vi "Emballage_BDD_GPAO_V_ARTICLE_NOS_ARTtoINDEX.vi"(0 "codification":string, 5 "suffixe":string, 9 "clc_designation":string, 11 "error in (no error)":errorcluster) -> (2 "SUFFIXE":string, 3 "NB_PIECE_EMB":string, 4 "données":string[][](array[string]), 6 "id_article":string, 8 "INDICE_REV":string, 10 "REVIS_SUFF":string, 14 "pce_non_annule":bool, 15 "error out":errorcluster)   [LabVIEW 2020]
uses:
  Modules/FS/60_FS_Controles/60_FS_SetGet.ctl
  <vilib>/addons/database/Connection.llb/DB Tools Open Connec (Path).vi
  <vilib>/addons/database/Connection.llb/Conn Execute.vi
  <vilib>/addons/database/Recordset.llb/Rec Fetch Recordset Data (R).vi
  <vilib>/addons/database/Recordset.llb/Rec Destroy - Connection.vi
  <vilib>/addons/database/NI_Database_API.lvlib
panel:
  out "données 2":string[][](array[string])
  out "ENR_ANNULE":string
  in  "Liste multicolonne":i32(listbox)
  out "columns 2":string[](array[string])
  out "Requète":string
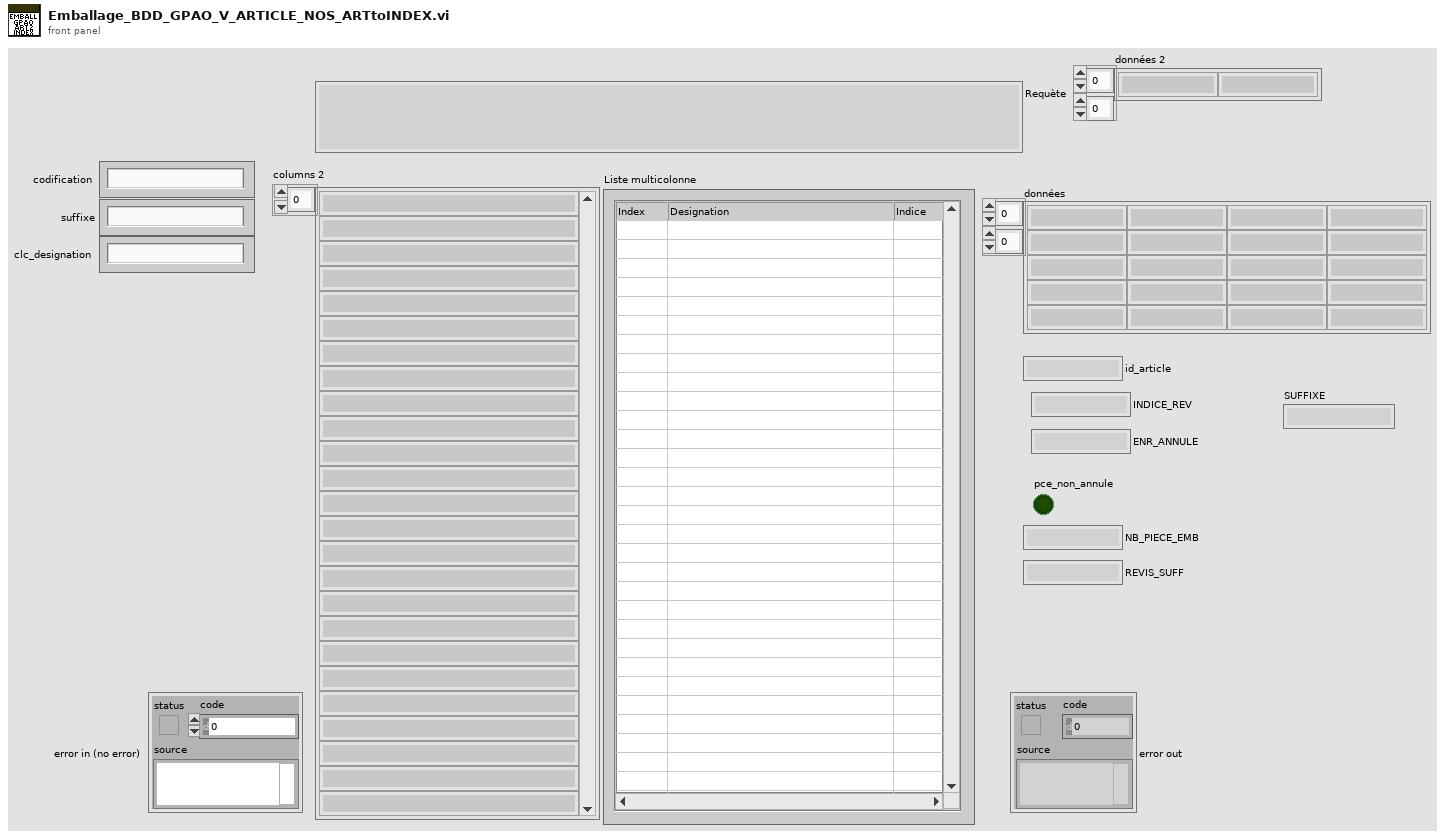
[diagram p1: front panel]
types:
  T1 = typedef "60_FS_SetGet.ctl" = enum16{"set", "get"}
  T2 = typedef "60_FS_CLT_Chemins.ctl" = cluster{"Racine_local":path, "Racine_reseau":path, "Racine_Support_Application":path, "Fichier_Journalisation":path, "Connexion_BDD_VSX":path, "Connexion_BDD_PLZ":path}
  T3 = typedef "NI_Database_API.lvlib/Conn ObjectReference.ctl" = refnum<k1>
  T4 = typedef "NI_Database_API.lvlib/Rec ObjectReference.ctl" = refnum<k1>
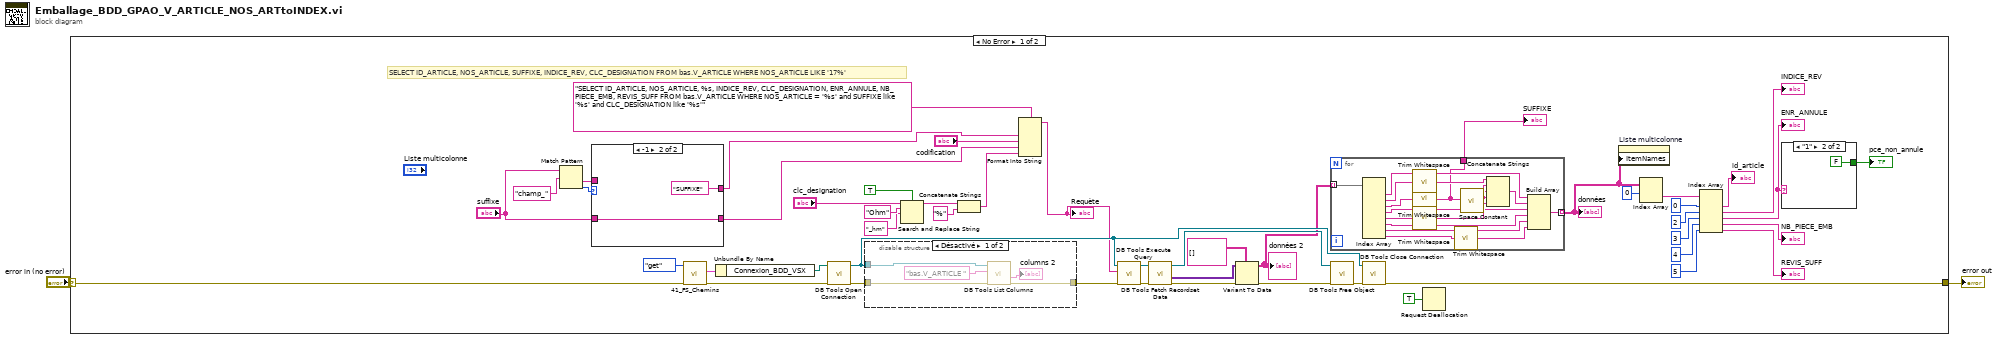
[diagram p0: block diagram]
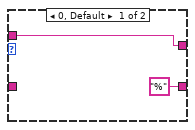
[diagram p2: hidden frame]
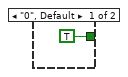
[diagram p3: hidden frame]
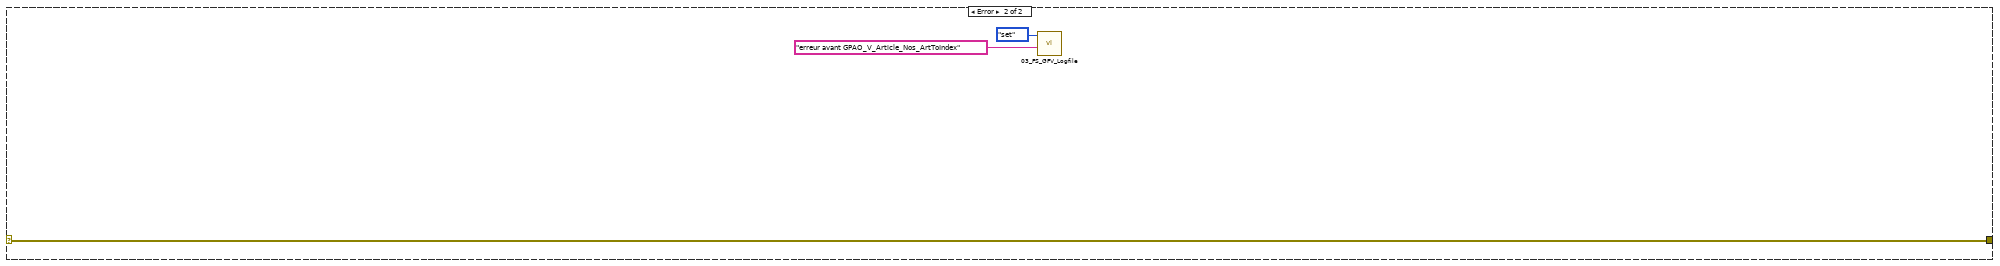
[diagram p5: hidden frame]
diagram:
  n1 = case shown="No Error" "error in (no error)" {
    selector: "error in (no error)" -> [w17 w83]
    tunnel: [w16 w83] -> w1
    frame No Error {
      # "SELECT ID_ARTICLE, NOS_ARTICLE, SUFFIXE, INDICE_REV, CLC_DESIGNATION FROM bas.V_ARTICLE WHERE NOS_ARTICLE LIKE '17%'"
      n2 = Match Pattern(string="suffixe", regular expression="champ_" ("expression régulière")) -> (after substring=w12:string, offset past match=w11:i32)  [unwired: 1 in, 2 out]
      n3 = case shown="-1" w11 {
        tunnel: [w54 "SUFFIXE"] -> w6
        tunnel: w12 -> [w54 _]
        tunnel: ["%" ("suffixe") w55] -> w4
        tunnel: "suffixe" -> [_ w55]
        frame 0, Default {
        }
        frame -1 {
        }
      }
      n4 = call "41_FS_Chemins.vi"("error in (no error)"=w17, "SetGet"=60_FS_SetGet."get") -> ("error out"=w50:errorcluster, "CLT_Chemins_out"=w51:T2)  [unwired: 8 in]
      n5 = Unbundle By Name(w51) -> ("Connexion_BDD_VSX"=w41:path)
      n6 = call-poly <vilib>:"DB Tools Open Connection.vi"("error in (no error)"=w50, "connection information"=w41) -> ("error out"=w39:errorcluster, "connection reference"=w40:T3)  [unwired: 6 in]
      n7 = disable-structure shown="Désactivé" {
        disable-tunnel: w40 -> [w79 _]
        disable-tunnel: w39 -> [w76 w80]
        disable-tunnel: [w75 w80] -> w38
        frame Disabled {
          n8 = call <vilib>:"DB Tools List Columns.vi"("error in (no error)"=w76, "table"="bas.V_ARTICLE " ("Table"), "connection reference"=w79) -> ("error out"=w75:errorcluster, "columns"=→"columns 2":string[])  [unwired: 1 in, 2 out]
        }
        frame Enabled {
        }
      }
      n9 = Search and Replace String(case sensitive?=TRUE ("ignorer la casse ? (F)"), input string="clc_designation", search string="Ohm" ("chaîne recherchée"), replace string="_hm" ("chaîne de remplacement (\"\")")) -> (result string=w14:string)  [unwired: 4 in, 3 out]
      n10 = Concatenate Strings(w14, "%" ("chaîne")) -> (w8:string)
      n11 = Format Into String(format string="SELECT ID_ARTICLE, NOS_ARTICLE, %s, INDICE_REV, CLC_DESIGNATION, ENR_ANNULE, NB_PIECE_EMB, REVIS_SUFF FROM bas.V_ARTICLE WHERE NOS_ARTICLE = '%s' and SUFFIXE like '%s' and CLC_DESIGNATION like '%s'" ("Requète"), w6, "codification", w4, w8) -> (resulting string=w9:string)  [unwired: 2 in, 1 out]
      "Requète" <- w9
      n12 = call-poly <vilib>:"DB Tools Execute Query.vi"("error in (no error)"=w38, "SQL query"=w9, "connection reference"=w40) -> ("error out"=w49:errorcluster, "recordset reference"=w48:T4)  [unwired: 5 in]
      n13 = call-poly <vilib>:"DB Tools Fetch Recordset Data.vi"("error in (no error)"=w49, "recordset reference"=w48) -> ("error out"=w45:errorcluster, "recordset data"=w46:variant[][], "recordset reference out"=w43:T4)  [unwired: 3 in]
      n14 = Variant To Data(error in=w45, type=string[][] [] ("Chaînes []"), Variant=w46) -> (data=w36:string[][], error out=w44:errorcluster)
      "données 2" <- w36
      n15 = for {
        tunnel: w36 -> [w74] mode=indexing
        tunnel: [w66] -> w31 mode=indexing
        tunnel: [w59] -> w5
        n16 = Index Array(array=w74) -> (element #1=w73:string, element #2=w71:string, element #3=w60:string, element #4=w64:string, element #5=w69:string, element #6=w65:string, element #7=w63:string, element #8=w62:string)  [unwired: 8 in]
        n17 = call <vilib>:"Trim Whitespace.vi"("string"=w71) -> ("trimmed string"=w70:string)  [unwired: 1 in]
        n18 = call <vilib>:"Trim Whitespace.vi"("string"=w60) -> ("trimmed string"=w59:string)  [unwired: 1 in]
        n19 = call <vilib>:"Trim Whitespace.vi"("string"=w69) -> ("trimmed string"=w68:string)  [unwired: 1 in]
        n20 = call <vilib>:"Trim Whitespace.vi"("string"=w62) -> ("trimmed string"=w61:string)  [unwired: 1 in]
        n21 = call <vilib>:"Space Constant.vi"() -> ("String"=w67:string)
        n22 = Concatenate Strings(w70, w67, w59, w67, w68) -> (w72:string)
        n23 = Build Array(w73, w72, w64, w65, w63, w61) -> (w66:string[])
      }
      "données" <- w31
      "SUFFIXE" <- w5
      n24 = call-poly <vilib>:"DB Tools Free Object.vi"("error in (no error)"=w44, "recordset reference"=w43) -> ("error out"=w42:errorcluster)  [unwired: 8 in, 1 out]
      n25 = call <vilib>:"DB Tools Close Connection.vi"("error in (no error)"=w42, "connection reference"=w40) -> ("error out"=w16:errorcluster)  [unwired: 5 in]
      n26 = Request Deallocation(TRUE ("flag")) -> ()
      n27 = property on="Liste multicolonne" class="MCListbox (strict)"("ItemNames"=w31) -> ()  [unwired: 2 in, 2 out]
      n28 = Index Array(array=w31, index (row)=0 ("indice (ligne)")) -> (element=w29:string[])  [unwired: 1 in]
      n29 = Index Array(array=w29, index #1=0 ("indice"), index #2=2 ("indice"), index #3=3 ("indice"), index #4=4 ("indice"), index #5=5 ("indice")) -> (element #1=→"id_article":string, element #2=→"INDICE_REV":string, element #3=w23:string, element #4=→"NB_PIECE_EMB":string, element #5=→"REVIS_SUFF":string)
      "ENR_ANNULE" <- w23
      n30 = case shown="\"1\"" w23 {
        tunnel: [TRUE FALSE] -> w22
        frame "0", Default {
        }
        frame "1" {
        }
      }
      "pce_non_annule" <- w22
    }
    frame Error {
      n31 = call "03_FS_GFV_Logfile.vi"("Chaîne"="erreur avant GPAO_V_Article_Nos_ArtToIndex", "States"=60_FS_SetGet."set") -> ()  [unwired: 8 in, 2 out]
    }
  }
  "error out" <- w1
